vi "MoveXYRelative.vi"(8 "error in (no error)":errorcluster, 9 "Y":dbl, 10 "X":dbl, 11 "connection ID":refnum<k5>) -> (0 "error out":errorcluster, 3 "connection ID 2":refnum<k5>)   [LabVIEW 2019]
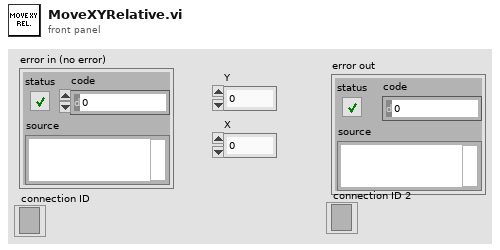
[diagram p1: front panel]
types:
  T1 = enum16{"Standard", "Buffered", "CRLF", "Immediate"}
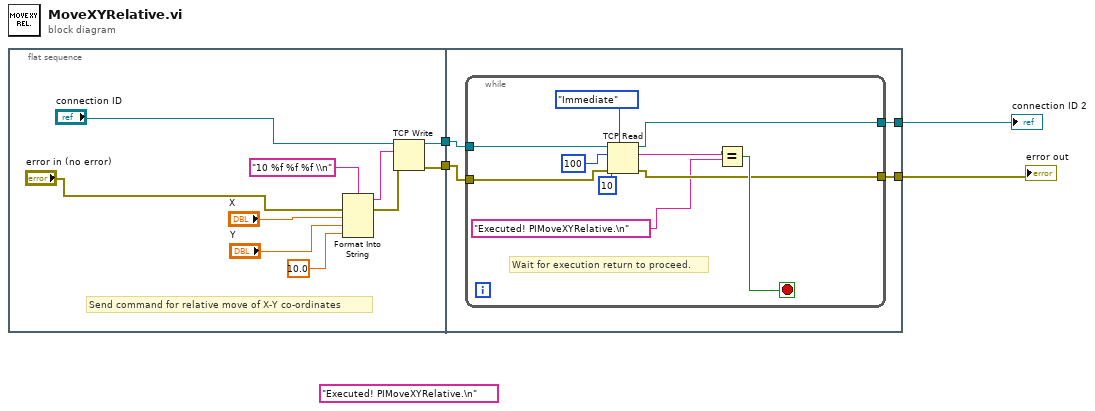
[diagram p0: block diagram]
diagram:
  (unwired) "Executed! PIMoveXYRelative.\n"
  n1 = flat-sequence {
    tunnel: [w8] -> w4
    tunnel: [w7] -> w3
    tunnel: w4 -> [w17]
    tunnel: w3 -> [w18]
    tunnel: [w16] -> w2
    tunnel: [w15] -> w1
    frame #0 {
      # "Send command for relative move of X-Y co-ordinates"
      n2 = Format Into String(format string="10 %f %f %f \\n", error in="error in (no error)", "X", "Y", 10.0 ("input 3")) -> (resulting string=w10:string, error out=w9:errorcluster)  [unwired: 1 in]
      n3 = TCP Write(connection ID="connection ID", data in=w10, error in (no error)=w9) -> (connection ID out=w8:refnum<k5>, error out=w7:errorcluster)  [unwired: 1 in, 1 out]
    }
    frame #1 {
      n4 = while {
        tunnel: w18 -> [w26]
        tunnel: [w22] -> w16
        tunnel: [w21] -> w15
        tunnel: w17 -> [w19]
        stop <- w23 stop-if-true
        # "Wait for execution return to proceed."
        n5 = TCP Read(connection ID=w19, bytes to read=100, error in (no error)=w26, 7:T1."Immediate" ("mode (standard)"), 9:10 ("timeout ms (25000)")) -> (connection ID out=w21:refnum<k5>, data out=w24:string, error out=w22:errorcluster)
        n6 = Equal?(x=w24, y="Executed! PIMoveXYRelative.\n") -> (x = y?=w23:bool)
      }
    }
  }
  "error out" <- w2
  "connection ID 2" <- w1
